vi "Read Index.vi"(8 "error in (no error)":errorcluster, 11 "Local Bus_Access_Int in":refnum<class "Local Bus_Int.lvclass">) -> (0 "error out":errorcluster, 2 "Index":i32, 3 "Local Bus_Access_Int out":refnum<class "Local Bus_Int.lvclass">)   [LabVIEW 2021, in "Local Bus_Int.lvclass"]
uses:
  Local Bus_Int.lvclass
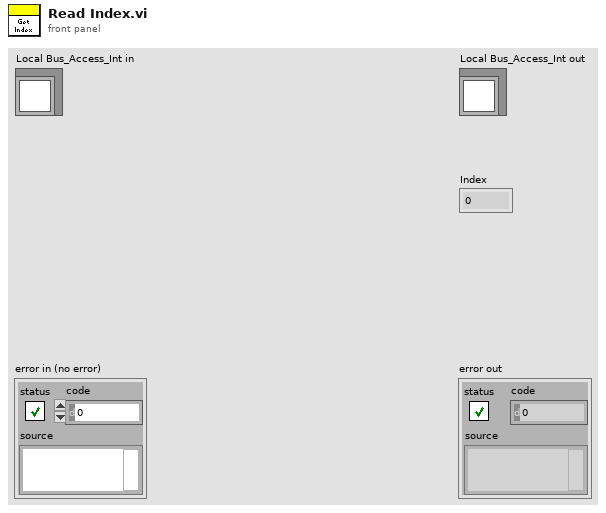
[diagram p1: front panel]
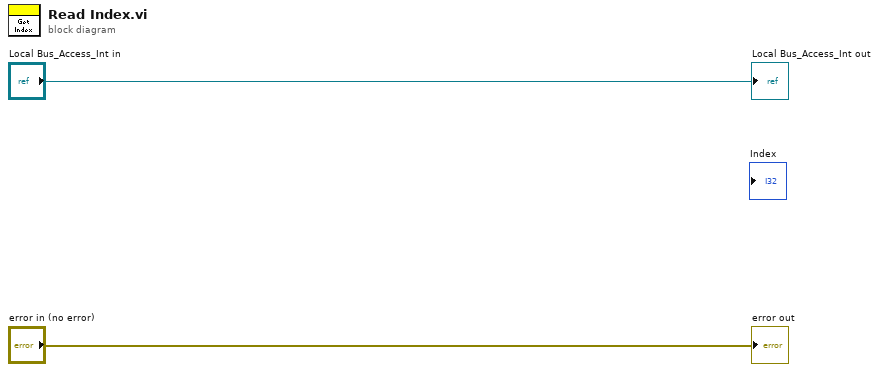
[diagram p0: block diagram]
diagram:
  "error out" <- "error in (no error)"
  "Local Bus_Access_Int out" <- "Local Bus_Access_Int in"
